vi "pcfs_close_devices.vi"(8 "error in (no error)":errorcluster, 11 "pcfs in":refnum<class "pcfs.lvclass">) -> (0 "error out":errorcluster, 3 "pcfs out":refnum<class "pcfs.lvclass">)   [LabVIEW 2015, in "pcfs.lvclass"]
uses:
  pcfs.lvclass
  pcfs.lvclass/pcfs.ctl
  UI/panel_class/panel.lvclass
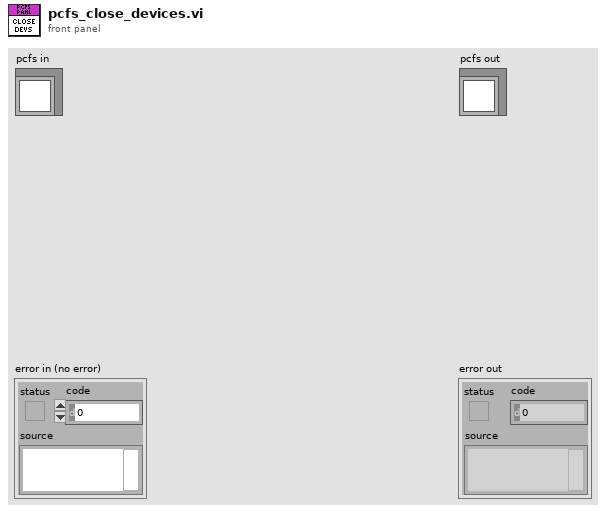
[diagram p1: front panel]
types:
  T1 = typedef "hardware_caller_queue_numbers.ctl" = enum16{"stage1", "stage2", "experiment", "detector"}
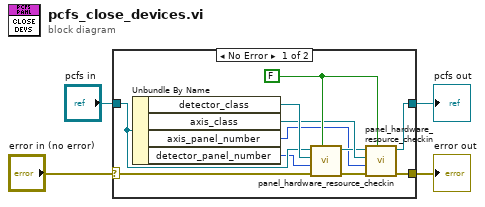
[diagram p0: block diagram]
diagram:
  n1 = case shown="No Error" "error in (no error)" {
    selector: "error in (no error)" -> [w9 w17]
    tunnel: [w8 w17] -> w3
    tunnel: [w7 w16] -> w1
    tunnel: "pcfs in" -> [w12 w16]
    frame No Error {
      w15 = FALSE ("Self")
      n2 = Unbundle By Name(w12) -> ("detector_class"=w14:refnum<class "detector.lvclass">, "axis_class"=w13:refnum<class "Stage.lvclass">, "axis_panel_number"=w6:T1, "detector_panel_number"=w5:T1)
      n3 = call "panel_hardware_resource_checkin.vi"("Self"=w15, "error in (no error)"=w9, "panel_number"=w5, "hardware.lvclass"=w14, "panel in"=w12) -> ("error out"=w10:errorcluster, "panel out"=w11:refnum<class "pcfs.lvclass">)  [unwired: 5 in]
      n4 = call "panel_hardware_resource_checkin.vi"("Self"=w15, "error in (no error)"=w10, "panel_number"=w6, "hardware.lvclass"=w13, "panel in"=w11) -> ("error out"=w8:errorcluster, "panel out"=w7:refnum<class "pcfs.lvclass">)  [unwired: 5 in]
    }
    frame Error {
    }
  }
  "error out" <- w3
  "pcfs out" <- w1
